vi "Get Driver Version.vi"(8 "error in (no error)":errorcluster) -> (0 "error out":errorcluster, 2 "Library Version":string)   [LabVIEW 2019, in "D2XX-lv.lvlib"]
doc: "This function returns D2XX DLL version number."
uses:
  D2XX-lv.lvlib
  <instrlib>/_D2XX/D2XX/D2XX.lvlib
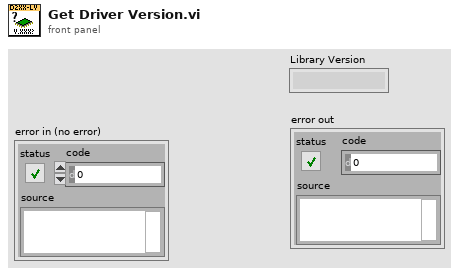
[diagram p1: front panel]
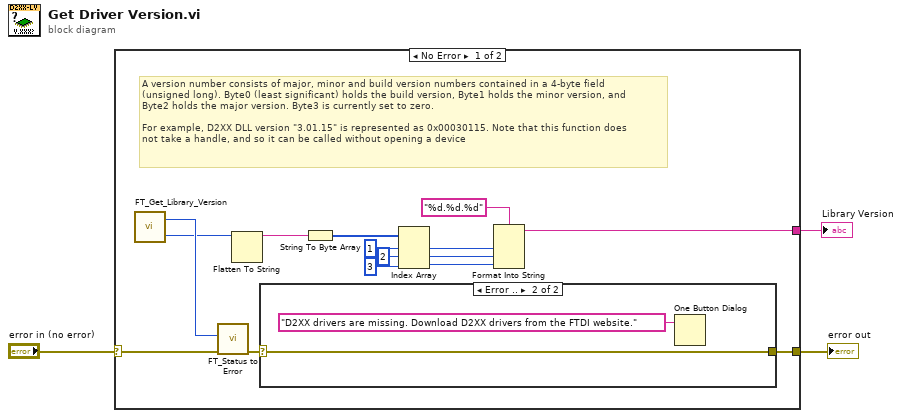
[diagram p0: block diagram]
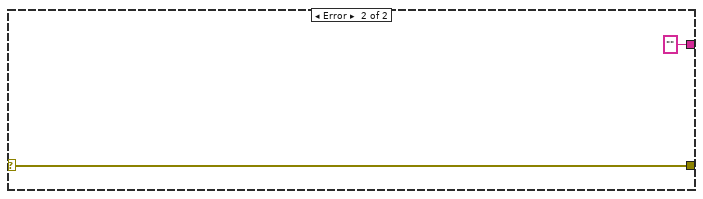
[diagram p3: hidden frame]
diagram:
  n1 = case shown="No Error" "error in (no error)" {
    selector: "error in (no error)" -> [w18 w23]
    tunnel: [w15 w23] -> w2
    tunnel: [w4 ""] -> w1
    frame No Error {
      # "A version number consists of major, minor and build version numbers contained in a 4-byte field\n(unsigned long). Byte0 (least significant) holds the build version, Byte1 holds the minor version, and\nByte2 holds the major version. Byte3 is currently set to zero.\n\nFor example, D2XX DLL version \"3.01.15\" is represented as 0x00030115. Note that this function does\nnot take a handle, and so it can be called without opening a device"
      n2 = call <instrlib>:"FT_Get_Library_Version.vi"() -> ("Library Version"=w14:u32, "FT_Status"=w17:u32)
      n3 = call "FT_Status to Error.vi"("error in (no error)"=w18, "FT_Status"=w17) -> ("error out"=w16:errorcluster)  [unwired: 9 in]
      n4 = Flatten To String(anything=w14) -> (data string=w13:string)  [unwired: 3 in, 2 out]
      n5 = case shown="Error .." w16 {
        selector: w16 -> [w19 w20]
        tunnel: [w19 w20] -> w15
        frame No Error {
        }
        frame Error {
          n6 = One Button Dialog(message="D2XX drivers are missing. Download D2XX drivers from the FTDI website.") -> ()  [unwired: 1 in, 1 out]
        }
      }
      n7 = String To Byte Array(string=w13) -> (unsigned byte array=w8:u8[])
      n8 = Index Array(array=w8, index #1=1 ("index"), index #2=2 ("index"), index #3=3 ("index")) -> (element #1=w11:u8, element #2=w9:u8, element #3=w10:u8)
      n9 = Format Into String(format string="%d.%d.%d", w11, w9, w10) -> (resulting string=w4:string)  [unwired: 2 in, 1 out]
    }
    frame Error {
    }
  }
  "error out" <- w2
  "Library Version" <- w1
